vi "Manual Mode.vi"() -> ()   [LabVIEW 2015]
uses:
  Common/Buffers/Snapshot/Snapshot.lvclass
  CAN Communication/Oil/Oil.lvclass
panel:
  in  "RMP In":dbl=100.0
  out "Test Leak Rate (PSI/s)":dbl format="%#.2f"
  out "Temp (C)":dbl format="%#.2f"
  out "MIO (%)":dbl format="%#.2f"
  out "Oil Pressure (PSI)":dbl format="%#.2f"
  out "DAQ Errors":errorcluster
  out "Oil Board Errors":errorcluster
  out "Control Block Error":errorcluster
  in  "SV1":bool
  in  "OK Button":bool
  in  "Oil Pump":bool
  in  "3WV2":bool
  in  "3WV1":bool
  in  "Vacuum":bool
  in  "GV2":bool
  in  "GV1":bool
  in  "SV2":bool
  out "Test Pressure (PSI)":dbl format="%#.2f"
  # "Manual Mode"
  # "Live Data Display"
  # "Oil Board"
  # "Oil Valve Control"
  # "Control Block"
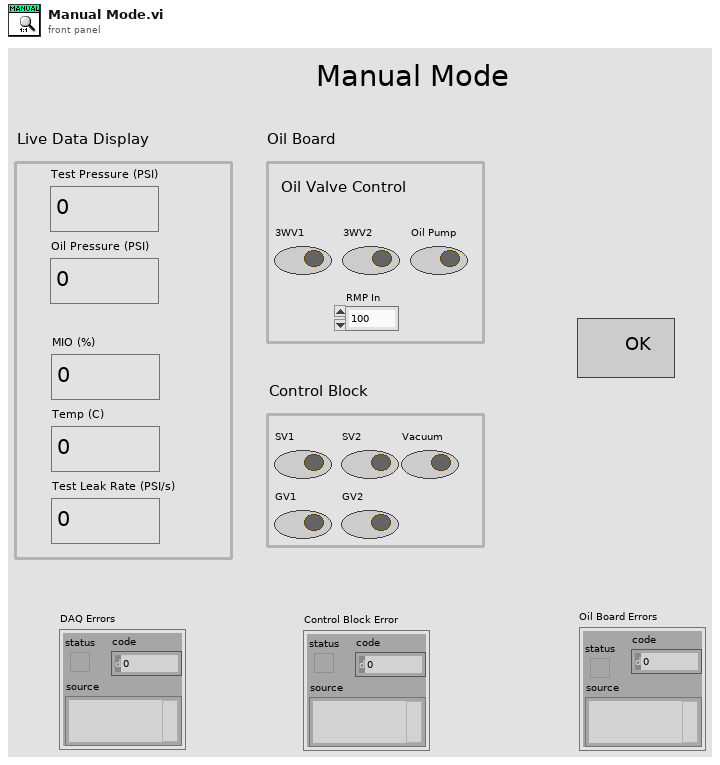
[diagram p1: front panel]
types:
  T1 = typedef "Oil.lvclass/Session Handle.ctl" = refnum<data-value>
  T2 = typedef "Snapshot.lvclass/Session Handle.ctl" = refnum<data-value>
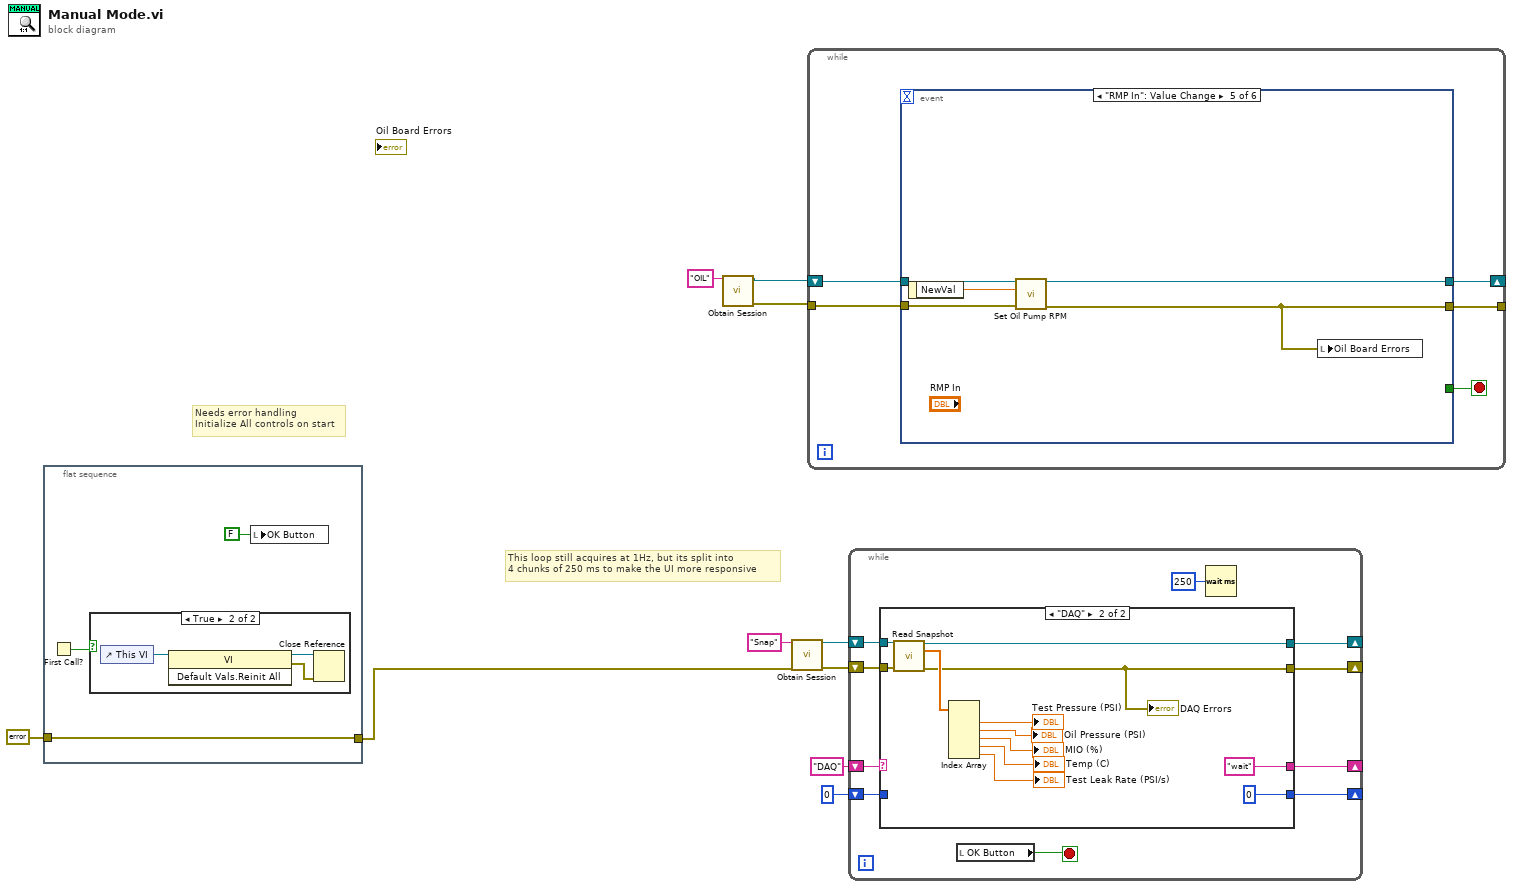
[diagram p0: block diagram]
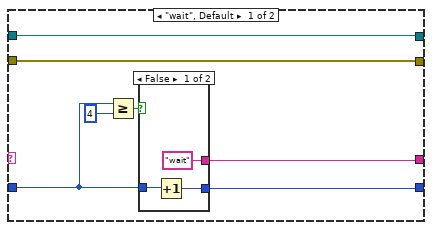
[diagram p2: hidden frame]
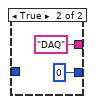
[diagram p3: hidden frame]
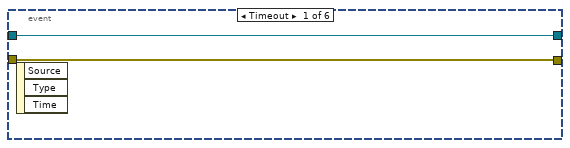
[diagram p5: hidden frame]
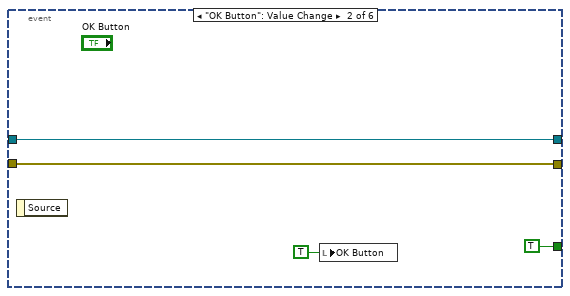
[diagram p6: hidden frame]
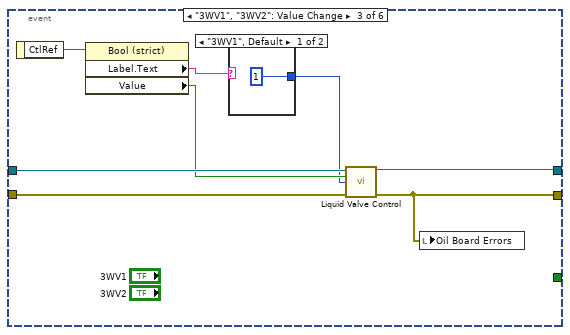
[diagram p7: hidden frame]
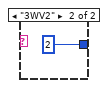
[diagram p8: hidden frame]
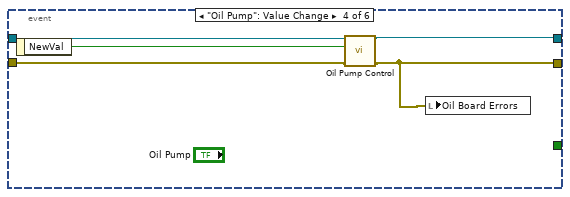
[diagram p9: hidden frame]
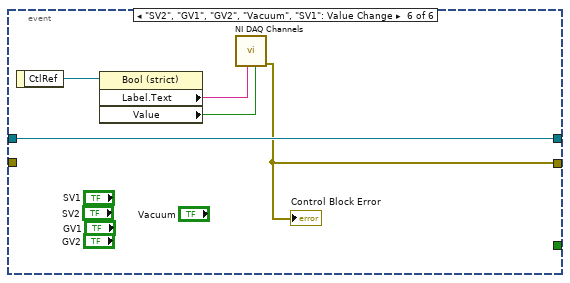
[diagram p10: hidden frame]
diagram:
  # "This loop still acquires at 1Hz, but its split into\n4 chunks of 250 ms to make the UI more responsive"
  # "Needs error handling\nInitialize All controls on start"
  n1 = flat-sequence {
    tunnel: errorcluster {"status"=FALSE, "code"=0, "source"=""} ("error in (no error)") -> [w12]
    tunnel: [w12] -> w4
    frame #0 {
      n2 = First Call?() -> (First Call?: T/F=w11:bool)
      n3 = case shown="True" w11 {
        frame False {
        }
        frame True {
          n4 = control-ref of="This VI"() -> (w16:refnum<vi>)
          n5 = invoke class="VI" method="Default Vals.Reinit All"(reference=w16) -> (reference out=w14:refnum<vi>, error out=w15:errorcluster)  [unwired: 2 in, 1 out]
          n6 = Close Reference(reference=w14, error in (no error)=w15) -> ()  [unwired: 1 out]
        }
      }
      n7 = local write "OK Button"(FALSE ("OK Button")) -> ()
    }
  }
  n8 = call "Obtain Session.vi"("Session  Name ()"="OIL") -> ("Session Handle"=w2:T1, "error out"=w1:errorcluster)  [unwired: 13 in]
  n9 = call "Obtain Session.vi"("Session  Name ()"="Snap", "error in (no error)"=w4) -> ("Session Handle"=w8:T2, "error out"=w7:errorcluster)  [unwired: 12 in]
  n10 = while {
    shift-right: [w19] -> _
    shift-left: w2 -> [w21]
    tunnel: w1 -> [w20]
    tunnel: [w18] -> _
    stop <- w17 stop-if-true
    n11 = event shown="[4] \"RMP In\": Value Change" {
      selector: _ -> [_ _ _ _ _ _]
      dyn-events: _ -> [_ _ _ _ _ _]
      timeout: _ -> [_ _ _ _ _ _]
      tunnel: w21 -> [w23 w27 w34 w41 w47 w52]
      tunnel: w20 -> [w22 w26 w33 w40 w44 _]
      tunnel: [w23 w27 w29 w42 w46 w52] -> w19
      tunnel: [w22 w26 w28 w38 w43 w48] -> w18
      tunnel: [_ TRUE ("OK Button") _ _ _ _] -> w17
      event Timeout {
        n12 = event-data() -> ()  [unwired: 1 in, 3 out]
      }
      event "OK Button": Value Change {
        n13 = event-data() -> ()  [unwired: 1 in, 1 out]
        n14 = local write "OK Button"(TRUE ("OK Button")) -> ()
      }
      event "3WV1", "3WV2": Value Change {
        n15 = event-data() -> ("CtlRef"=w35:refnum<vi>)  [unwired: 1 in]
        n16 = property class="Bool (strict)"(reference=w35) -> ("Label.Text"=w31:string, "Value"=w32:bool)  [unwired: 1 in, 2 out]
        n17 = case shown="\"3WV1\", Default" w31 {
          tunnel: [1 ("Valve") 2 ("Valve")] -> w30
          frame "3WV1", Default {
          }
          frame "3WV2" {
          }
        }
        n18 = call "Liquid Valve Control.vi"("Session Handle in"=w34, "On?"=w32, "Valve"=w30, "error in (no error)"=w33) -> ("Session Handle out"=w29:T1, "error out"=w28:errorcluster)  [unwired: 8 in, 2 out]
        n19 = local write "Oil Board Errors"(w28) -> ()
      }
      event "Oil Pump": Value Change {
        n20 = event-data() -> ("NewVal"=w39:bool)  [unwired: 1 in]
        n21 = call "Oil Pump Control.vi"("Session Handle in"=w41, "On?"=w39, "error in (no error)"=w40) -> ("Session Handle out"=w42:T1, "error out"=w38:errorcluster)  [unwired: 9 in, 2 out]
        n22 = local write "Oil Board Errors"(w38) -> ()
      }
      event "RMP In": Value Change {
        n23 = event-data() -> ("NewVal"=w45:dbl)  [unwired: 1 in]
        n24 = call "Set Oil Pump RPM.vi"("Session Handle in"=w47, "RPM"=w45, "error in (no error)"=w44) -> ("Session Handle out"=w46:T1, "error out"=w43:errorcluster)  [unwired: 9 in, 2 out]
        n25 = local write "Oil Board Errors"(w43) -> ()
      }
      event "SV2", "GV1", "GV2", "Vacuum", "SV1": Value Change {
        n26 = event-data() -> ("CtlRef"=w51:refnum<vi>)  [unwired: 1 in]
        n27 = property class="Bool (strict)"(reference=w51) -> ("Label.Text"=w50:string, "Value"=w49:bool)  [unwired: 1 in, 2 out]
        n28 = call "NI DAQ Channels.vi"("Control"=w49, "Channel"=w50) -> ("error out"=w48:errorcluster)  [unwired: 8 in, 1 out]
        "Control Block Error" <- w48
      }
    }
  }
  n29 = while {
    shift-right: [w59] -> _
    shift-left: w8 -> [w60]
    shift-right: [w58] -> _
    shift-left: w7 -> [w61]
    shift-right: [w56] -> _
    shift-left: "DAQ" -> [w57]
    shift-right: [w55] -> _
    shift-left: 0 -> [w54]
    stop <- w62 stop-if-true
    n30 = case shown="\"DAQ\"" w57 {
      tunnel: w61 -> [w68 w86]
      tunnel: w60 -> [w69 w85]
      tunnel: [w69 w84] -> w59
      tunnel: [w68 w79] -> w58
      tunnel: [w63 "wait"] -> w56
      tunnel: [w64 0] -> w55
      tunnel: w54 -> [w65 _]
      frame "wait", Default {
        n31 = Greater Or Equal?(x=w65, y=4) -> (x >= y?=w66:bool)
        n32 = case shown="False" w66 {
          tunnel: w65 -> [w72 _]
          tunnel: [w71 0] -> w64
          tunnel: ["wait" "DAQ"] -> w63
          frame False {
            n33 = Increment(x=w72) -> (x+1=w71:i32)
          }
          frame True {
          }
        }
      }
      frame "DAQ" {
        n34 = call "Read Snapshot.vi"("Session Handle in"=w85, "error in (no error)"=w86) -> ("Session Handle out"=w84:T2, "Buffer"=w83:dbl[], "error out"=w79:errorcluster)  [unwired: 11 in]
        "DAQ Errors" <- w79
        n35 = Index Array(array=w83) -> (element #1=→"Test Pressure (PSI)":dbl, element #2=→"Oil Pressure (PSI)":dbl, element #3=→"MIO (%)":dbl, element #4=→"Temp (C)":dbl, element #5=→"Test Leak Rate (PSI/s)":dbl)  [unwired: 5 in]
      }
    }
    n36 = local read "OK Button"() -> (w62:bool)
    n37 = Wait (ms)(milliseconds to wait=u32 250) -> ()  [unwired: 1 out]
  }
